vi "Build Major Frame Instructions.vi"(7 "Virtual Memory Unit in":refnum<class "Virtual Memory Unit.lvclass">, 8 "error in (no error)":errorcluster, 9 "Minor Frame Pointers":T1 {"HP Async Address" format="%04x"; "Next Frame Address" format="%04x"; "SubRoutine Address" format="%04x"}, 10 "Starting Address":u16 format="%04x", 11 "Minor Frame in":refnum<class "Minor Frame.lvclass">) -> (0 "error out":errorcluster, 1 "Already Config'd":bool, 2 "Next Available Address":u16 format="%04x", 3 "Minor Frame out":refnum<class "Minor Frame.lvclass">, 5 "Virtual Memory Unit out":refnum<class "Virtual Memory Unit.lvclass">)   [LabVIEW 2020, in "BCI-1553 API.lvlib" / "Minor Frame.lvclass"]
doc: "<DO NOT CALL>\n\nInserts the commands into the Major Frame instruction list for the Minor Frame execution. Every Minor Frame is followed by a call to the check for the next Minor Frame subroutine."
uses:
  Minor Frame.lvclass
  Dependencies/Virtual Memory Unit/Virtual Memory Unit.lvclass
  TypeDefs/Minor Frame Pointers.ctl
  TypeDefs/BC Op Codes - Verbose.ctl
  TypeDefs/BC Condition Codes.ctl
  Minor Frame.lvclass/Minor Frame.ctl
  BCI-1553 API.lvlib
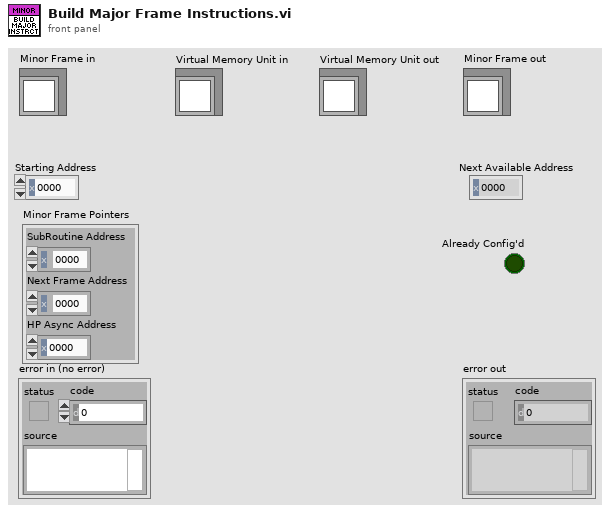
[diagram p1: front panel]
types:
  T1 = typedef "BCI-1553 API.lvlib/Minor Frame Pointers.ctl" = cluster{"SubRoutine Address":u16, "Next Frame Address":u16, "HP Async Address":u16}
  T2 = typedef "BCI-1553 API.lvlib/BC Condition Codes.ctl" = enum16{"GP0 == 1 || LT", "GP1 == 1 || NE", "GP2 == 1", "GP3 == 1", "GP4 == 1", "GP5 == 1", "GP6 == 1", "GP7 == 1", "NORESP", "FMTERR", "GOODBLOCK", "MSKSTATSET", "BADMSG", "1RETRY", "2RETRY", "ALWAYS"}
  T3 = typedef "BCI-1553 API.lvlib/BC Op Codes - Verbose.ctl" = enum16{"EXECUTE MSG", "EXECUTE MSG GO", "JUMP", "CALL SUBROUTINE", "RETURN", "INTERRUPT REQUEST", "HALT", "DELAY", "WAIT FRAME TIMER = 0", "COMPARE FRAME TIMER", "COMPARE MSG TIMER", "LOAD TIME TAG CTR", "LOAD TIME TAG CTR HI", "LOAD FRAME TIMER", "START FRAME TIMER", "PUSH TIME TAG COUNT", "PUSH TIME TAG COUNT HI", "PUSH TIME TAG COUNT BOTH", "PUSH BLOCK STATUS WORD", "PUSH CURRENT VALUE", "PUSH INDIRECT", "WAIT EXT TRIGGER", "EXECUTE AND FLIP", "EXECUTE, FLIP, GO", "WRITE VALUE TO WMI", "WRITE VALUE TO MEM", "DECREMENT RAM, SKIP", "FLAG"}
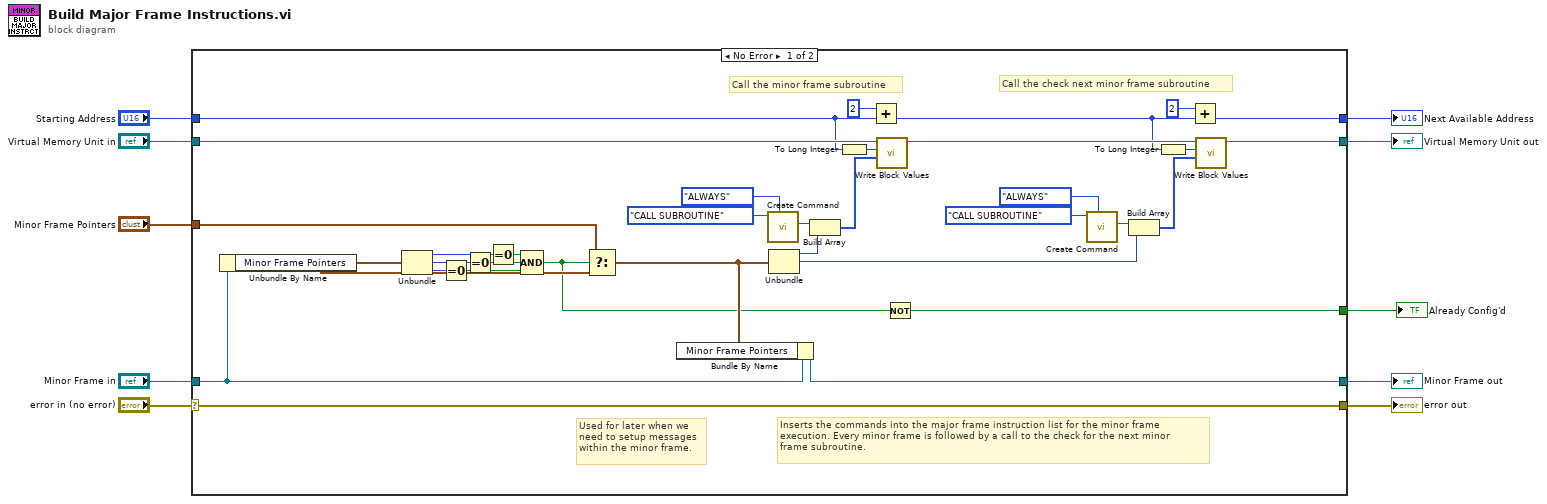
[diagram p0: block diagram]
diagram:
  n1 = case shown="No Error" "error in (no error)" {
    selector: "error in (no error)" -> [w44 w48]
    tunnel: [w44 w48] -> w9
    tunnel: [w23 w47] -> w7
    tunnel: "Minor Frame in" -> [w19 w47]
    tunnel: "Virtual Memory Unit in" -> [w43 w45]
    tunnel: "Starting Address" -> [w29 w46]
    tunnel: "Minor Frame Pointers" -> [w14 _]
    tunnel: [w30 w45] -> w3
    tunnel: [w26 w46] -> w2
    tunnel: [w11 _] -> w1
    frame No Error {
      # "Used for later when we\nneed to setup messages\nwithin the minor frame."
      # "Inserts the commands into the major frame instruction list for the minor frame\nexecution. Every minor frame is followed by a call to the check for the next minor\nframe subroutine."
      # "Call the check next minor frame subroutine"
      # "Call the minor frame subroutine"
      n2 = Unbundle By Name(w19) -> ("Minor Frame Pointers"=w15:T1)
      n3 = Unbundle(w15) -> ("SubRoutine Address"=w22:u16, "Next Frame Address"=w21:u16, "HP Async Address"=w20:u16)
      n4 = Equal To 0?(x=w20) -> (x = 0?=w16:bool)
      n5 = Equal To 0?(x=w21) -> (x = 0?=w17:bool)
      n6 = Equal To 0?(x=w22) -> (x = 0?=w18:bool)
      n7 = Compound Arithmetic op=AND(w18, w17, w16) -> (w12:bool)
      n8 = Select(t=w14, s=w12, f=w15) -> (s? t:f=w13:T1)
      n9 = Bundle By Name(cluster=w19, "Minor Frame Pointers"=w13) -> (w23:refnum<class "Minor Frame.lvclass">)
      n10 = call "Create Command.vi"("Condition"=BC_Condition_Codes."ALWAYS", "Op Code"=BC_Op_Codes_-_Verbose."CALL SUBROUTINE") -> ("Instruction"=w39:u16)  [unwired: 8 in, 1 out]
      n11 = Unbundle(w13) -> ("SubRoutine Address"=w38:u16, "Next Frame Address"=w24:u16)  [unwired: 1 out]
      n12 = Build Array(w39, w38) -> (w37:u16[])
      n13 = To Long Integer(number=w29) -> (32bit integer=w42:i32)
      n14 = Add(x=u16 2, y=w29) -> (x+y=w28:u16)
      n15 = call "Write Block Values.vi"("Write Block"=w37, "Start Index"=w42, "Virtual Memory Unit in"=w43) -> ("Virtual Memory Unit out"=w31:refnum<class "Virtual Memory Unit.lvclass">)  [unwired: 7 in, 1 out]
      n16 = Not(x=w12) -> (.not. x?=w11:bool)
      n17 = call "Create Command.vi"("Condition"=BC_Condition_Codes."ALWAYS", "Op Code"=BC_Op_Codes_-_Verbose."CALL SUBROUTINE") -> ("Instruction"=w35:u16)  [unwired: 8 in, 1 out]
      n18 = Build Array(w35, w24) -> (w36:u16[])
      n19 = To Long Integer(number=w28) -> (32bit integer=w32:i32)
      n20 = Add(x=u16 2, y=w28) -> (x+y=w26:u16)
      n21 = call "Write Block Values.vi"("Write Block"=w36, "Start Index"=w32, "Virtual Memory Unit in"=w31) -> ("Virtual Memory Unit out"=w30:refnum<class "Virtual Memory Unit.lvclass">)  [unwired: 7 in, 1 out]
    }
    frame Error {
    }
  }
  "error out" <- w9
  "Minor Frame out" <- w7
  "Next Available Address" <- w2
  "Virtual Memory Unit out" <- w3
  "Already Config'd" <- w1
